vi "索引.vi"() -> ()   [LabVIEW 2018]
panel:
  out "元素":dbl
  in  "停止":bool
  in  "索引 列":i32
  in  "索引 行":dbl
  in  "数组":dbl[][](array[numeric])
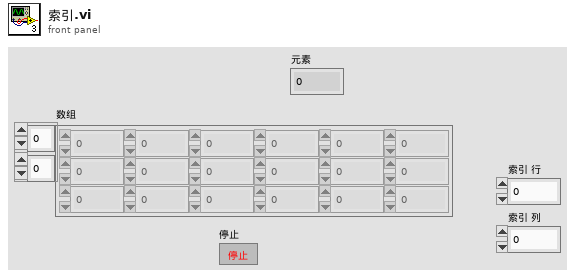
[diagram p1: front panel]
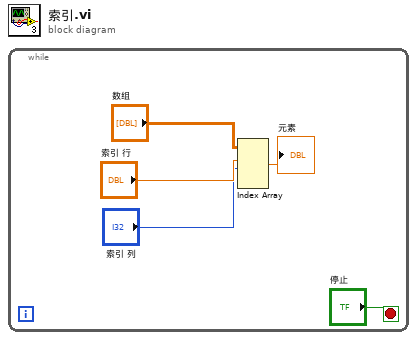
[diagram p0: block diagram]
diagram:
  n1 = while {
    stop <- "停止" stop-if-true
    n2 = Index Array(array="数组", index (row) #1="索引 行", index (col) #1="索引 列") -> (element #1=→"元素":dbl)  [unwired: 2 in, 1 out]
  }
